vi "Pade get coeff_test.vi"(8 "x array":dbl[](array[numeric])=[0.0, 0.05, 0.1, 0.15, 0.2, 0.25, 0.3, 0.35, 0.4, 0.45, 0.5, 0.55, 0.6, 0.65, 0.7, 0.75, 0.8, 0.85, 0.9, 0.95, 1.0, 1.05, 1.1, 1.15, 1.2, 1.25, 1.3, 1.35, 1.4, 1.45, 1.5, 1.55, 1.6, 1.65, 1.7, 1.75, 1.8, 1.85, 1.9, 1.95, 2.0, 2.05, 2.1, 2.15, 2.2, 2.25, 2.3, 2.35, 2.4, 2.45, 2.5, 2.55, 2.6, 2.65, 2.7, 2.75, 2.8, 2.85, 2.9, 2.95, 3.0, 3.05, 3.1, 3.15, 3.2, 3.25, 3.3, 3.35, 3.4, 3.45, 3.5, 3.55, 3.6, 3.65, 3.7, 3.75, 3.8, 3.85, 3.9, 3.95, 4.0, 4.05, 4.1, 4.15, 4.2, 4.25, 4.3, 4.35, 4.4, 4.45, 4.5, 4.55, 4.6, 4.65, 4.7, 4.75, 4.8, 4.85, 4.9, 4.95], 9 "n":i32=6, 10 "m":i32=6, 11 "Derivatives":dbl[](array[numeric])=[0.0, 1.0, 0.0, -1.0, 0.0, 1.0, 0.0, -1.0, 0.0, 1.0, 0.0, -1.0, 0.0] format="%.2f") -> (0 "error":i32, 1 "Pade_mn array":dbl[](array[numeric]), 2 "Denominator":dbl[](array[numeric])=[1.0, -4.8693611902790253e-14, 0.0367101138425998, -1.4269963388078193e-15, 0.0006886010742634833, -3.4269662069482143e-17, 7.261928768281087e-06] format="%.6f", 3 "Numerator":dbl[](array[numeric])=[-2.636779683484747e-16, 0.999999999999999, -4.771877337717001e-14, -0.12995655282406612, 6.1201044232461754e-15, 0.0029035821004963977, 3.95516952522712e-16] format="%.6f")   [LabVIEW 2021]
uses:
  <vilib>/Analysis/7linalg.llb/Solve Linear Equations (single right hand).vi
  <vilib>/Analysis/2dsp.llb/1D Convolution (DBL).vi
  <vilib>/Analysis/baseanly.llb/Solve Linear Equations By Cholesky.vi
  <vilib>/Analysis/baseanly.llb/Real Matrix to Compact Array.vi
  <vilib>/Analysis/baseanly.llb/Real Compact Tri-Matrix Linear Eqs.vi
  <vilib>/Analysis/7linalg.llb/Solve Linear Eqs (General).vi
  <vilib>/Analysis/7linalg.llb/Solve Linear Eqs (Gen, single right hand).vi
  <vilib>/Analysis/NI_AALPro.lvlib
panel:
  out "XY Graph":cluster{dbl[], dbl[]}(graph)={[0.0, 0.05, 0.1, 0.15, 0.2, 0.25, 0.3, 0.35, 0.4, 0.45, 0.5, 0.55, 0.6, 0.65, 0.7, 0.75, 0.8, 0.85, 0.9, 0.95, 1.0, 1.05, 1.1, 1.15, 1.2, 1.25, 1.3, 1.35, 1.4, 1.45, 1.5, 1.55, 1.6, 1.65, 1.7, 1.75, 1.8, 1.85, 1.9, 1.95, 2.0, 2.05, 2.1, 2.15, 2.2, 2.25, 2.3, 2.35, 2.4, 2.45, 2.5, 2.55, 2.6, 2.65, 2.7, 2.75, 2.8, 2.85, 2.9, 2.95, 3.0, 3.05, 3.1, 3.15, 3.2, 3.25, 3.3, 3.35, 3.4, 3.45, 3.5, 3.55, 3.6, 3.65, 3.7, 3.75, 3.8, 3.85, 3.9, 3.95, 4.0, 4.05, 4.1, 4.15, 4.2, 4.25, 4.3, 4.35, 4.4, 4.45, 4.5, 4.55, 4.6, 4.65, 4.7, 4.75, 4.8, 4.85, 4.9, 4.95], [-2.636779683484747e-16, 0.049979169270678026, 0.09983341664682781, 0.14943813247359883, 0.19866933079506088, 0.24740395925452255, 0.2955202066613392, 0.34289780745545123, 0.3894183423086521, 0.43496553411123906, 0.4794255386042388, 0.5226872289307838, 0.5646424733954211, 0.6051864057371278, 0.6442176872405311, 0.6816387600302671, 0.7173560909154885, 0.7512804051752239, 0.7833269097005189, 0.8134155049360173, 0.8414709850918147, 0.8674232261259477, 0.8912073610287395, 0.9127639419723369, 0.9320390889220492, 0.9489846243405102, 0.9635581936511405, 0.9757233711637952, 0.985449751202827, 0.99271302421592, 0.9974950376809675, 0.9997838416678083, 0.9995737189517965, 0.9968651996168121, 0.9916650601263816, 0.9839863068829448, 0.9738481443368974, 0.961275927748777, 0.9463011007496813, 0.9289611178866963, 0.909299352381568, 0.887364989372026, 0.8632129049459083, 0.8369035313184335, 0.8085027085424966, 0.778081523180579, 0.745716134404667, 0.7114875880272782, 0.6754816190022114, 0.6377884429677866, 0.5985025374380167, 0.5577224132781615, 0.5155503771303799, 0.47209228548251453, 0.4274572910983113, 0.3817575825504395, 0.33510811761843295, 0.28762635133194536, 0.23943195945543963, 0.1906465582234417, 0.14139342114575315, 0.09179719370936472, 0.04198360680823775, -0.007920810266502827, -0.05778901644509982, -0.10749374428032799, -0.15690778331316085, -0.2059042605958098, -0.25435691757920104, -0.30214038258920534, -0.3491304381361734, -0.3952042823256159, -0.44024078366392155, -0.48412072858189625, -0.5267270610303902, -0.5679451135362568, -0.6076628291432045, -0.6457709737005501, -0.682163338003299, -0.7167369293291433, -0.7493921519616514, -0.7800329763339376, -0.808567096473154, -0.8349060754730361, -0.8589654787692051, -0.8806649950396828, -0.89992854460098, -0.9166843752177068, -0.9308651452909754, -0.9424079944373466, -0.9512546015157698, -0.957351230204429, -0.9606487622725798, -0.9611027187340224, -0.958673269108676, -0.9533252290566373, -0.9450280466848421, -0.9337557778600667, -0.9194870508931661, -0.9022050209881741]}
  # "m >= n\n# of derivatives = m+n+1"
  # "Example: f(x)=sin (x)+1.23\nDerivatives: (1.23,1, 0, -1, 0, 1, ...) total 6+6+1=13 (upto 12th derivative)\nm: 6\n n: 6"
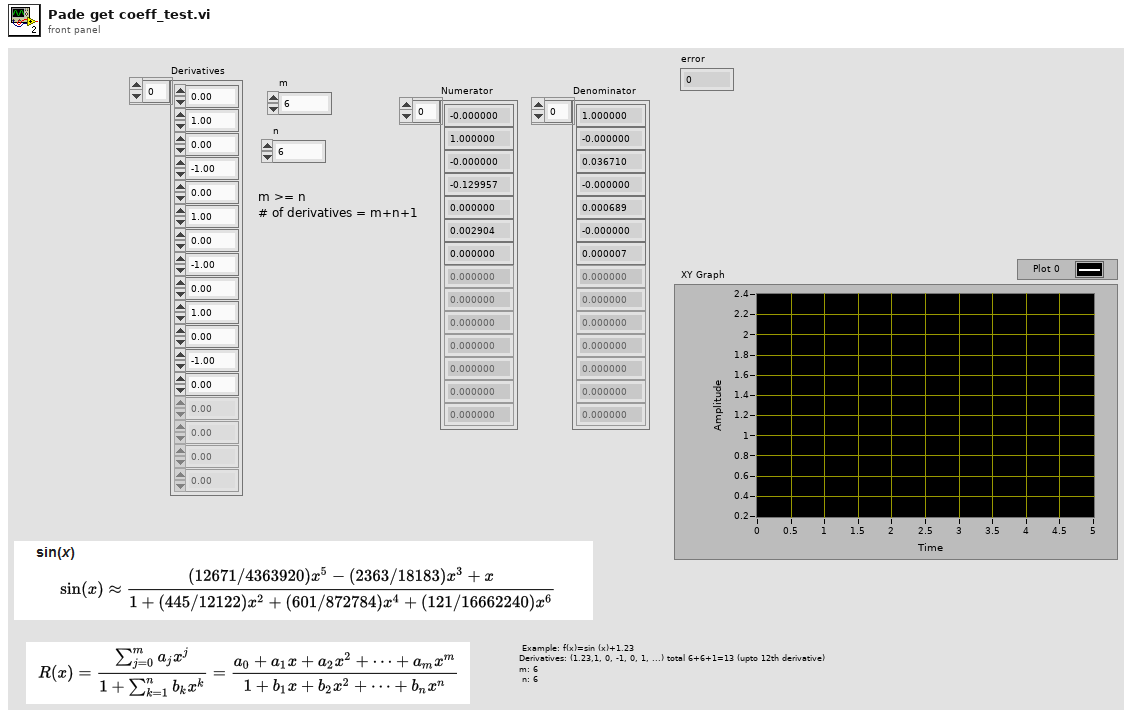
[diagram p1: front panel]
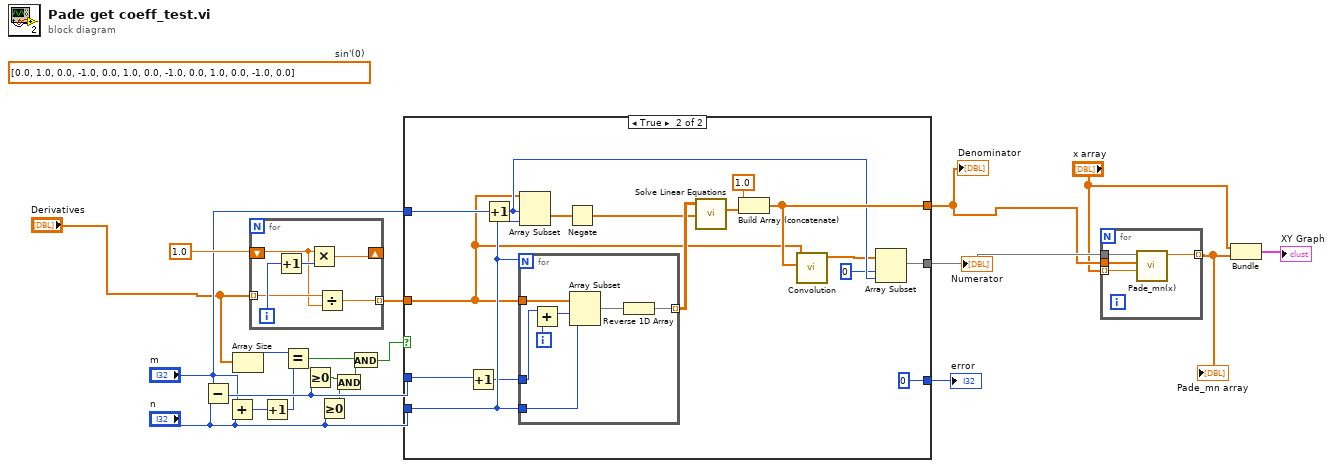
[diagram p0: block diagram]
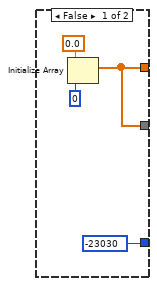
[diagram p2: hidden frame]
diagram:
  (unwired) dbl[] [0.0, 1.0, 0.0, -1.0, 0.0, 1.0, 0.0, -1.0, 0.0, 1.0, 0.0, -1.0, 0.0]  # sin'(0)
  n1 = Subtract(x="m", y="n") -> (x-y=w20:i32)
  n2 = Add(x="m", y="n") -> (x+y=w12:i32)
  n3 = Array Size(array="Derivatives") -> (size(s)=w8:i32)
  n4 = for {
    shift-right: [w26] -> _
    shift-left: 1.0 -> [w22]
    tunnel: "Derivatives" -> [w23] mode=indexing
    tunnel: [w21] -> w15 mode=indexing
    i -> [w25]
    n5 = Increment(x=w25) -> (x+1=w24:i32)
    n6 = Multiply(x=w22, y=w24) -> (x*y=w26:dbl)
    n7 = Divide(x=w23, y=w22) -> (x/y=w21:dbl)
  }
  n8 = Increment(x=w12) -> (x+1=w7:i32)
  n9 = Equal?(x=w8, y=w7) -> (x = y?=w11:bool)
  n10 = Greater Or Equal To 0?(x=w20) -> (x >= 0?=w19:bool)
  n11 = Greater Or Equal To 0?(x="n") -> (x >= 0?=w18:bool)
  n12 = And(x=w19, y=w18) -> (x .and. y?=w10:bool)
  n13 = And(x=w11, y=w10) -> (x .and. y?=w9:bool)
  n14 = case shown="True" w9 {
    tunnel: [w28 w46] -> w5
    tunnel: [w28 w45] -> w6
    tunnel: "m" -> [_ w37]
    tunnel: "n" -> [_ w36]
    tunnel: w20 -> [_ w34]
    tunnel: [-23030 0] -> w17
    tunnel: w15 -> [_ w31]
    frame False {
      n15 = Initialize Array(0.0, 0) -> (w28:dbl[])
    }
    frame True {
      n16 = Increment(x=w34) -> (x+1=w35:i32)
      n17 = Increment(x=w37) -> (x+1=w44:i32)
      n18 = for {
        N: w36 -> [_]
        tunnel: w31 -> [w53]
        tunnel: w36 -> [w52]
        tunnel: w35 -> [w51]
        tunnel: [w47] -> w39 mode=indexing
        i -> [w50]
        n19 = Add(x=w51, y=w50) -> (x+y=w49:i32)
        n20 = Array Subset(array=w53, index=w49, length=w52) -> (w48:dbl[])
        n21 = Reverse 1D Array(array=w48) -> (reversed array=w47:dbl[])
      }
      n22 = Array Subset(array=w31, index=w44, length=w36) -> (w38:dbl[])
      n23 = Negate(x=w38) -> (-x=w33:dbl[])
      n24 = call-poly <vilib>:"Solve Linear Equations.vi"("Known Vector"=w33, "Input Matrix"=w39) -> ("Solution Vector"=w40:dbl[])  [unwired: 1 in, 1 out]
      n25 = Build Array (concatenate)(1.0, w40) -> (w46:dbl[])
      n26 = call-poly <vilib>:"Convolution.vi"("Y"=w46, "X"=w31) -> ("X * Y"=w42:dbl[])  [unwired: 8 in, 1 out]
      n27 = Array Subset(array=w42, index=0, length=w44) -> (w45:dbl[])
    }
  }
  "Numerator" <- w6
  "Denominator" <- w5
  "error" <- w17
  n28 = for {
    tunnel: w6 -> [w57]
    tunnel: w5 -> [w56]
    tunnel: "x array" -> [w55] mode=indexing
    tunnel: [w54] -> w4 mode=indexing
    n29 = call "Pade_mn(x).vi"("x"=w55, "denominator"=w56, "numerator"=w57) -> ("Pm/n (x)"=w54:dbl)  [unwired: 8 in]
  }
  "Pade_mn array" <- w4
  n30 = Bundle("x array"="x array", w4) -> (→"XY Graph":cluster{"x array":dbl[], dbl[]})  [unwired: 1 in]
